vi "daqio_Switch_to_Device.vi"(7 "Device to switch to":T3, 8 "error in (no error)":errorcluster, 11 "daq.io type in":T1={"daq.io ref"=refnum, "daq.io API Base"="http://dashboard.daq.io/api/v1", "Device Type Key"="", "Device Key"="", "Account ID"="", "online"=TRUE, "SSL"=TRUE}) -> (0 "error out":errorcluster, 3 "daq.io type out":T1={"daq.io ref"=refnum, "daq.io API Base"="http://dashboard.daq.io/api/v1", "Device Type Key"="", "Device Key"="", "Account ID"="", "online"=TRUE, "SSL"=TRUE})   [LabVIEW 2013, in "daqio minimal.lvlib"]
doc: "This VI switches the active session to another device. All functions to create or update tags, events or time series data will now refer to the device.\n\nThis VI currently does not perform error checking on its inputs. When selecting devices or device types that do not exist, all following functions will generate errors."
uses:
  daqio minimal.lvlib
  _typedefs/daqio-Type.ctl
  <vilib>/httpClient/ClientHandle.ctl
  _typedefs/daqio-Device-Specifier.ctl
  <vilib>/httpClient/LabVIEWHTTPClient.lvlib
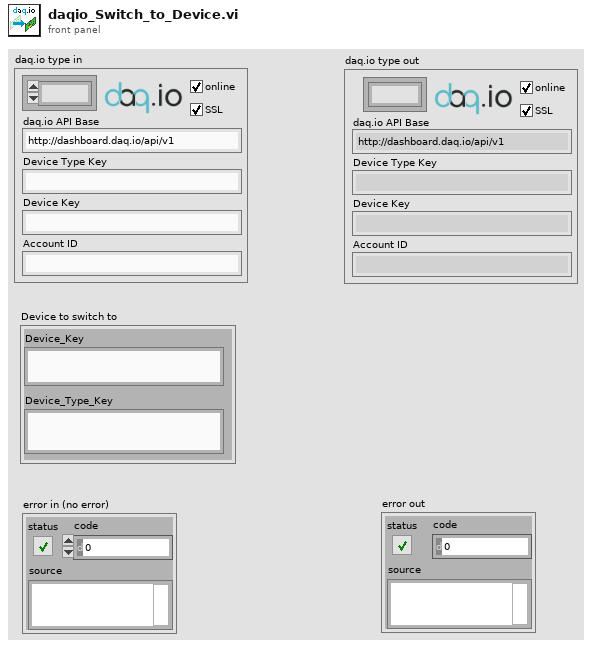
[diagram p1: front panel]
types:
  T1 = typedef "daqio minimal.lvlib/daqio-Type.ctl" = cluster{"daq.io ref":T2, "daq.io API Base":string, "Device Type Key":string, "Device Key":string, "Account ID":string, "online":bool, "SSL":bool}
  T2 = typedef "LabVIEWHTTPClient.lvlib/ClientHandle.ctl" = refnum<k1>
  T3 = typedef "daqio minimal.lvlib/daqio-Device-Specifier.ctl" = cluster{"Device_Key":string, "Device_Type_Key":string}
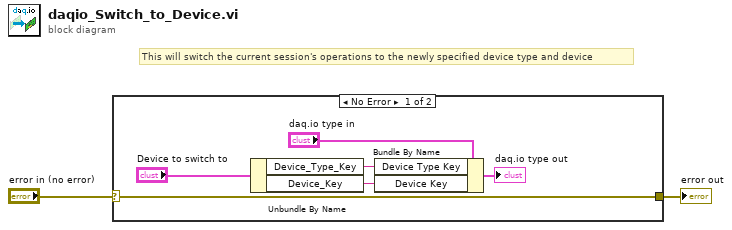
[diagram p0: block diagram]
diagram:
  # "This will switch the current session's operations to the newly specified device type and device"
  n1 = case shown="No Error" "error in (no error)" {
    selector: "error in (no error)" -> [w5 w9]
    tunnel: [w5 w9] -> w1
    frame No Error {
      n2 = Unbundle By Name("Device to switch to") -> ("Device_Type_Key"=w7:string, "Device_Key"=w8:string)
      n3 = Bundle By Name(cluster="daq.io type in", "Device Type Key"=w7, "Device Key"=w8) -> (→"daq.io type out":T1)
    }
    frame Error {
    }
  }
  "error out" <- w1
